vi "Power2Speed.vi"(10 "Power":dbl format="%#_13g") -> (2 "Speed":dbl format="%#_13g")   [LabVIEW 2017]
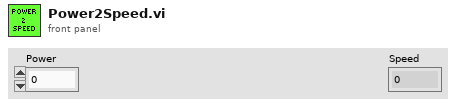
[diagram p1: front panel]
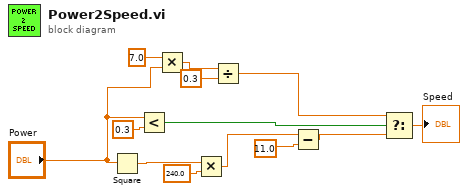
[diagram p0: block diagram]
diagram:
  n1 = Square(x="Power") -> (x^2=w2:dbl)
  n2 = Less?(x="Power", y=0.3) -> (x < y?=w12:bool)
  n3 = Multiply(x=7.0, y="Power") -> (x*y=w5:dbl)
  n4 = Multiply(x=w2, y=240.0) -> (x*y=w10:dbl)
  n5 = Divide(x=w5, y=0.3) -> (x/y=w3:dbl)
  n6 = Subtract(x=w10, y=11.0) -> (x-y=w1:dbl)
  n7 = Select(t=w3, s=w12, f=w1) -> (s? t:f=→"Speed":dbl)
